vi "test_VISA Protocol Factory.vi"(8 "error in (no error)":errorcluster, 11 "TestCase in":refnum<class "Instrument Addon Scripting API Protocol Factories Unit Tests.lvclass">) -> (0 "error out":errorcluster, 3 "TestCase out":refnum<class "Instrument Addon Scripting API Protocol Factories Unit Tests.lvclass">)   [LabVIEW 2018, in "Instrument Addon Scripting API Protocol Factories Unit Tests.lvclass"]
uses:
  Instrument Addon Scripting API Protocol Factories Unit Tests.lvclass
  VISA/VISA Settings.ctl
  VISA/VISA.lvclass
  VISA/VISA.lvclass/VISA.ctl
  VISA/Data Access/Read Append Write Termination Character.vi
  VISA/Data Access/Read Enable Termination Character.vi
  VISA/Data Access/Read Termination Character.vi
  VISA/Data Access/Read Timeout.vi
  VISA/Data Access/Read VISA Resource.vi
  <vilib>/addons/_JKI Toolkits/VI Tester/TestCase.llb/TestCase.lvclass
  C:/Program Files (x86)/National Instruments/LabVIEW 2018/vi.lib/addons/_JKI Toolkits/VI Tester/TestCase.llb/TestCase.lvclass
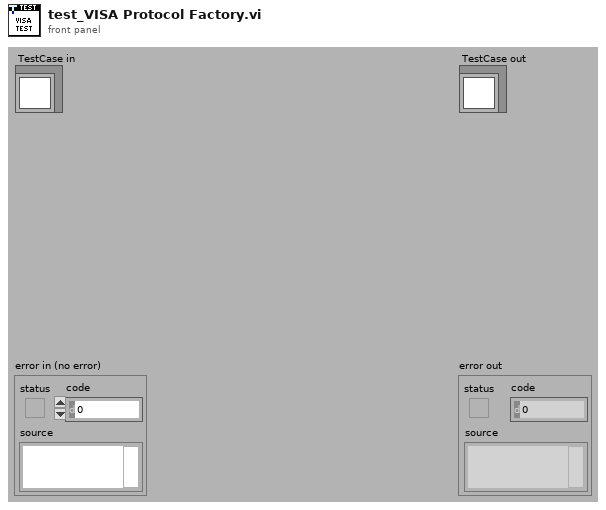
[diagram p1: front panel]
types:
  T1 = typedef "Protocols.lvlib/VISA.lvclass/VISA Settings.ctl" = cluster{"VISA Resource":string, "Enable Termination Character?":bool, "Termination Character":u8, "Timeout":u32, "Append Write Termination Character":bool}
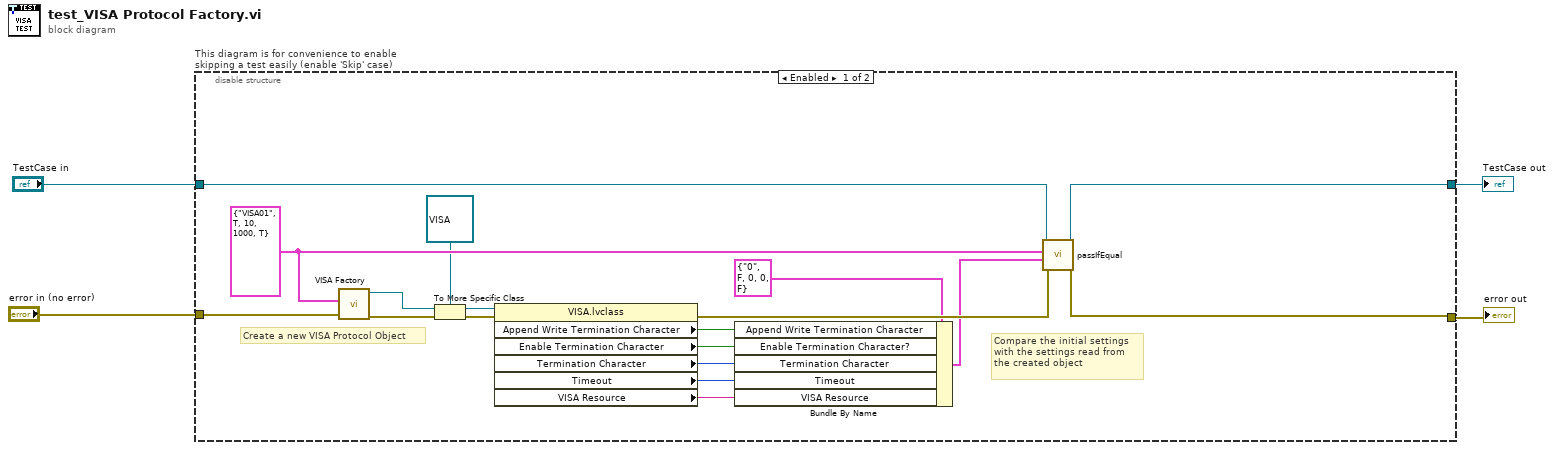
[diagram p0: block diagram]
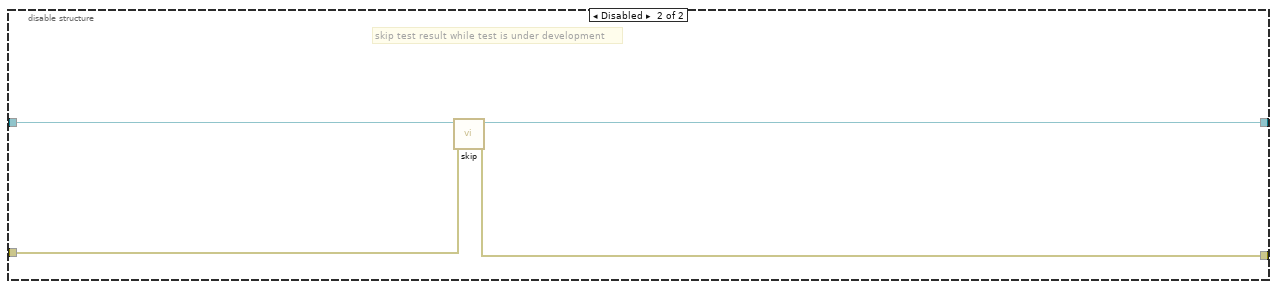
[diagram p2: hidden frame]
diagram:
  n1 = disable-structure "This diagram is for convenience to enable skipping a test easily (enable 'Skip' case)" shown="Enabled" {
    disable-tunnel: "TestCase in" -> [w22 w26]
    disable-tunnel: [w21 w24] -> w1
    disable-tunnel: [w20 w25] -> w3
    disable-tunnel: "error in (no error)" -> [w18 w23]
    frame Enabled {
      w17 = T1 {"VISA Resource"="VISA01", "Enable Termination Character?"=TRUE, "Termination Character"=10, "Timeout"=1000, "Append Write Termination Character"=TRUE} ("VISA Settings")
      # "Compare the initial settings \nwith the settings read from \nthe created object"
      # "Create a new VISA Protocol Object"
      n2 = call "VISA Factory.vi"("error in (no error)"=w18, "VISA settings"=w17) -> ("error out"=w8:errorcluster, "protocol out"=w9:refnum<class "Protocol Parent.lvclass">)  [unwired: 8 in]
      n3 = To More Specific Class(target class=refnum<class "VISA.lvclass"> refnum ("Protocols.lvlib:VISA.lvclass"), reference=w9, error in=w8) -> (specific class reference=w5:refnum<class "VISA.lvclass">, error out=w6:errorcluster)
      n4 = property class="VISA.lvclass"(reference=w5, error in=w6) -> (error out=w19:errorcluster, "Append Write Termination Character"=w15:bool, "Enable Termination Character"=w14:bool, "Termination Character"=w13:u8, "Timeout"=w12:u32, "VISA Resource"=w11:string)  [unwired: 1 out]
      n5 = Bundle By Name(cluster=T1 {"VISA Resource"="0", "Enable Termination Character?"=FALSE, "Termination Character"=0, "Timeout"=0, "Append Write Termination Character"=FALSE} ("VISA Settings"), "Append Write Termination Character"=w15, "Enable Termination Character?"=w14, "Termination Character"=w13, "Timeout"=w12, "VISA Resource"=w11) -> (w10:T1)
      n6 = call-dynamic "passIfEqual.vi"("error in (no error)"=w19, "y"=w10, "x"=w17, "TestCase in"=w22) -> ("error out"=w20:errorcluster, "TestCase out"=w21:refnum<class "Instrument Addon Scripting API Protocol Factories Unit Tests.lvclass">)  [unwired: 6 in]
    }
    frame Disabled {
      # "skip test result while test is under development"
      n7 = call <vilib>:"skip.vi"("error in (no error)"=w23, "TestCase in"=w26) -> ("error out"=w25:errorcluster, "TestCase out"=w24:refnum<class "Instrument Addon Scripting API Protocol Factories Unit Tests.lvclass">)  [unwired: 8 in]
    }
  }
  "error out" <- w3
  "TestCase out" <- w1
